vi "Set Line clock.vi"(11 "Refresh":bool) -> ()   [LabVIEW 2015]
uses:
  <vilib>/rvi/eio/common/nirviEmuTemplateMethod_errors.vi
  <vilib>/eio/EIONode/EIONode.xnode
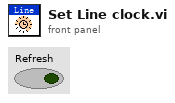
[diagram p1: front panel]
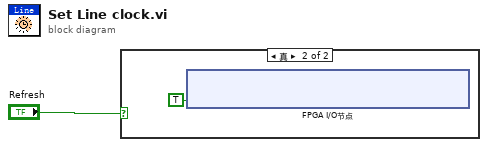
[diagram p0: block diagram]
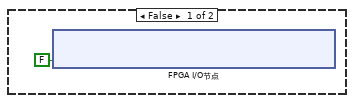
[diagram p2: hidden frame]
diagram:
  n1 = case shown="真" "Refresh" {
    frame False {
      n2 = xnode "FPGA I/O节点"("IO Module\\Line clock(DDCB_PFI2_WRITE)"=FALSE ("IO Module\\Line clock(DDCB_PFI2_WRITE)")) -> ()  [unwired: 1 in, 1 out]
    }
    frame True {
      n3 = xnode "FPGA I/O节点"("IO Module\\Line clock(DDCB_PFI2_WRITE)"=TRUE ("IO Module\\Line clock(DDCB_PFI2_WRITE)")) -> ()  [unwired: 1 in, 1 out]
    }
  }
